vi "attribute_write_double.vi"(5 "Repeated Capability":string, 7 "Attribute":T1={"Identifier"="", "Descriptive name"="", "Data Type"=enum."Integer 32", "Command"="", "Access"=2, "Range Table"="", "Read Callback"="", "Write Callback"="", "Range Callback"="", "Check Callback"="", "Rngtable Callback"="", "Coerce Callback"="", "Supported Models"="", "Instrument Options"="", "Repeated Capabilities"="", "Check Status Callback"="", "Index"=0, "Flag: OPC Wait"=FALSE, "Flag: Dont check status"=FALSE, "Flag: Cache Only"=FALSE} {"Access" items=["Read Only", "Write Only", "Read/Write"]}, 8 "error in":errorcluster, 10 "double in":dbl, 11 "VISA resource name":refnum<visa-resource-name>) -> (0 "error out":errorcluster, 3 "VISA resource name out":refnum<visa-resource-name>)   [LabVIEW 2014, in "rszvl_rsidr_core.lvlib"]
uses:
  rszvl_rsidr_core.lvlib
  type_Attribute.ctl
  type_Attribute_Data_Type.ctl
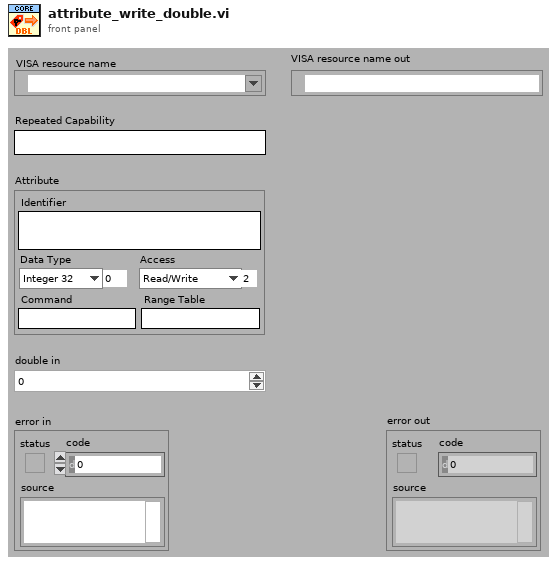
[diagram p1: front panel]
types:
  T1 = typedef "rszvl_rsidr_core.lvlib/type_Attribute.ctl" = cluster{"Identifier":string, "Descriptive name":string, "Data Type":T2, "Command":string, "Access":u16, "Range Table":string, "Read Callback":string, "Write Callback":string, "Range Callback":string, "Check Callback":string, "Rngtable Callback":string, "Coerce Callback":string, "Supported Models":string, "Instrument Options":string, "Repeated Capabilities":string, "Check Status Callback":string, "Index":i32, "Flag: OPC Wait":bool, "Flag: Dont check status":bool, "Flag: Cache Only":bool}
  T2 = typedef "rszvl_rsidr_core.lvlib/type_Attribute_Data_Type.ctl" = enum16{"Integer 32", "Double", "String", "Boolean", "None", "Integer 64"}
  T3 = typedef "rszvl_rsidr_core.lvlib/type_Session_Data.ctl" = cluster{"Instr type":string, "Instr type for err. msg.":string, "Installed Options":string[], "OPC Timeout":i32, "Query Instrument Status":bool, "Check Range":bool, "Check Options":bool, "Add LF to Write":bool, "Simulate":bool, "Logging":bool, "Logging params":variant, "Interface Type":enum16{"Unknown", "GPIB", "VXI", "GPIB_VXI", "ASRL", "PXI", "TCPIP", "USB", "SOCKET"}, "Fast Sweep":i32, "AdditionalFlags":i32, "WaitBeforeWrite":i32, "WaitBeforeRead":i32, "BinDataChunkSize":i64}
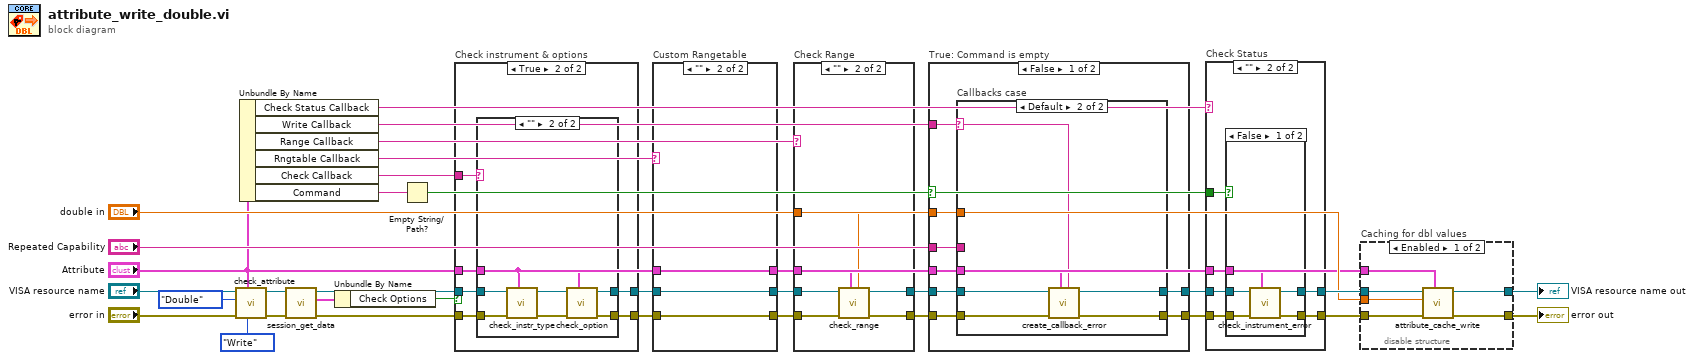
[diagram p0: block diagram]
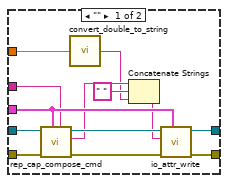
[diagram p2: hidden frame]
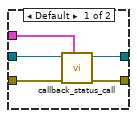
[diagram p4: hidden frame]
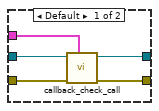
[diagram p7: hidden frame]
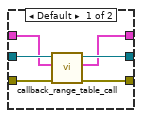
[diagram p8: hidden frame]
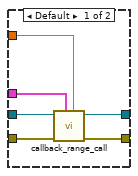
[diagram p9: hidden frame]
diagram:
  n1 = call "check_attribute.vi"("Access"=enum16{"Read", "Write"}."Write", "Attribute"="Attribute", "error in"="error in", "Data Type"=type_Attribute_Data_Type."Double", "VISA resource name"="VISA resource name") -> ("error out"=w9:errorcluster, "VISA resource name out"=w10:refnum<visa-resource-name>)  [unwired: 5 in]
  n2 = Unbundle By Name("Attribute") -> ("Check Status Callback"=w11:string, "Write Callback"=w12:string, "Range Callback"=w14:string, "Rngtable Callback"=w15:string, "Check Callback"=w13:string, "Command"=w1:string)
  n3 = call "session_get_data.vi"("error in"=w9, "VISA resource name"=w10) -> ("error out"=w7:errorcluster, "Session User Data out"=w4:T3, "VISA resource name out"=w8:refnum<visa-resource-name>)  [unwired: 7 in]
  n4 = Unbundle By Name(w4) -> ("Check Options"=w3:bool)
  n5 = Empty String/Path?(string/path=w1) -> (empty?=w33:bool)
  n6 = case "Check instrument & options" shown="True" w3 {
    tunnel: [w35 w41] -> w21
    tunnel: [w34 w40] -> w20
    tunnel: "Attribute" -> [_ w39]
    tunnel: w13 -> [_ w38]
    tunnel: w8 -> [w35 w37]
    tunnel: w7 -> [w34 w36]
    frame False {
    }
    frame True {
      n7 = case shown="\"\"" w38 {
        tunnel: [w45 w51] -> w41
        tunnel: [w43 w50] -> w40
        tunnel: w36 -> [w44 w49]
        tunnel: w39 -> [w42 w47]
        tunnel: w37 -> [w46 w48]
        frame Default {
          n8 = call "callback_check_call.vi"("Attribute"=w42, "error in"=w44, "VISA resource name"=w46) -> ("error out"=w43:errorcluster, "VISA resource name out"=w45:refnum<visa-resource-name>)  [unwired: 7 in]
        }
        frame "" {
          n9 = call "check_instr_type.vi"("Attribute"=w47, "error in"=w49, "VISA resource name"=w48) -> ("error out"=w53:errorcluster, "VISA resource name out"=w52:refnum<visa-resource-name>)  [unwired: 6 in, 1 out]
          n10 = call "check_option.vi"("Attribute"=w47, "error in"=w53, "VISA resource name"=w52) -> ("error out"=w50:errorcluster, "VISA resource name out"=w51:refnum<visa-resource-name>)  [unwired: 7 in]
        }
      }
    }
  }
  n11 = case "Custom Rangetable" shown="\"\"" w15 {
    tunnel: w21 -> [w59 w62]
    tunnel: w20 -> [w56 w61]
    tunnel: [w58 w62] -> w19
    tunnel: [w57 w61] -> w18
    tunnel: "Attribute" -> [w55 w60]
    tunnel: [w54 w60] -> w6
    frame Default {
      n12 = call "callback_range_table_call.vi"("error in"=w56, "Attribute in"=w55, "VISA resource name"=w59) -> ("error out"=w57:errorcluster, "Attribute out"=w54:T1, "VISA resource name out"=w58:refnum<visa-resource-name>)  [unwired: 6 in]
    }
    frame "" {
    }
  }
  n13 = case "Check Range" shown="\"\"" w14 {
    tunnel: w19 -> [w68 w74]
    tunnel: w18 -> [w65 w73]
    tunnel: w6 -> [w63 w70]
    tunnel: [w66 w72] -> w23
    tunnel: [w67 w71] -> w22
    tunnel: "double in" -> [w64 w69]
    frame Default {
      n14 = call "callback_range_call.vi"("Attribute Value"=w64, "Attribute"=w63, "error in"=w65, "VISA resource name"=w68) -> ("error out"=w66:errorcluster, "VISA resource name out"=w67:refnum<visa-resource-name>)  [unwired: 4 in, 2 out]
    }
    frame "" {
      n15 = call "check_range.vi"("Attribute Value"=w69, "Attribute"=w70, "error in"=w73, "VISA resource name"=w74) -> ("error out"=w72:errorcluster, "VISA resource name out"=w71:refnum<visa-resource-name>)  [unwired: 4 in, 2 out]
    }
  }
  n16 = case "True: Command is empty" shown="False" w33 {
    tunnel: "Repeated Capability" -> [w82 _]
    tunnel: w23 -> [w81 w102]
    tunnel: w22 -> [w80 w103]
    tunnel: "double in" -> [w79 _]
    tunnel: w6 -> [w78 _]
    tunnel: [w77 w103] -> w17
    tunnel: [w76 w102] -> w16
    tunnel: w12 -> [w75 _]
    frame False {
      n17 = case "Callbacks case" shown="Default" w75 {
        selector: w75 -> [_ w96]
        tunnel: w80 -> [w94 w100]
        tunnel: w81 -> [w92 w101]
        tunnel: w82 -> [w88 _]
        tunnel: [w91 w98] -> w77
        tunnel: [w90 w99] -> w76
        tunnel: w78 -> [w89 w97]
        tunnel: w79 -> [w83 _]
        frame "" {
          n18 = call "rep_cap_compose_cmd.vi"("Repeated Capability"=w88, "Attribute"=w89, "error in"=w92, "VISA resource name"=w94) -> ("error out"=w93:errorcluster, "Command out"=w87:string, "VISA resource name out"=w95:refnum<visa-resource-name>)  [unwired: 5 in]
          n19 = call "convert_double_to_string.vi"("double in"=w83) -> ("string out"=w84:string)  [unwired: 4 in]
          n20 = Concatenate Strings(w87, " " ("string"), w84) -> (w85:string)
          n21 = call "io_attr_write.vi"("Attribute"=w89, "error in"=w93, "write buffer"=w85, "VISA resource name"=w95) -> ("error out"=w90:errorcluster, "VISA resource name out"=w91:refnum<visa-resource-name>)  [unwired: 6 in]
        }
        frame Default {
          n22 = call "create_callback_error.vi"("Callback Name"=w96, "Attribute"=w97, "error in"=w101, "VISA resource name"=w100) -> ("error out"=w99:errorcluster, "VISA resource name out"=w98:refnum<visa-resource-name>)  [unwired: 6 in]
        }
      }
    }
    frame True {
    }
  }
  n23 = case "Check Status" shown="\"\"" w11 {
    tunnel: w16 -> [w108 w113]
    tunnel: [w107 w112] -> w32
    tunnel: [w106 w111] -> w31
    tunnel: w17 -> [w105 w114]
    tunnel: w6 -> [w104 w110]
    tunnel: w33 -> [_ w109]
    frame Default {
      n24 = call "callback_status_call.vi"("Attribute"=w104, "error in"=w108, "VISA resource name"=w105) -> ("error out"=w107:errorcluster, "VISA resource name out"=w106:refnum<visa-resource-name>)  [unwired: 7 in]
    }
    frame "" {
      n25 = case shown="False" w109 {
        tunnel: w114 -> [w119 w121]
        tunnel: w113 -> [w118 w120]
        tunnel: [w117 w120] -> w112
        tunnel: [w116 w121] -> w111
        tunnel: w110 -> [w115 _]
        frame False {
          n26 = call "check_instrument_error.vi"("Attribute"=w115, "error in"=w118, "VISA resource name"=w119) -> ("error out"=w117:errorcluster, "VISA resource name out"=w116:refnum<visa-resource-name>)  [unwired: 7 in]
        }
        frame True {
        }
      }
    }
  }
  n27 = disable-structure "Caching for dbl values" shown="Enabled" {
    disable-tunnel: [w127 w129] -> w27
    disable-tunnel: [w126 w128] -> w26
    disable-tunnel: w32 -> [w125 w128]
    disable-tunnel: w31 -> [w124 w129]
    disable-tunnel: "double in" -> [w123 _]
    disable-tunnel: "Attribute" -> [w122 _]
    frame Enabled {
      n28 = call "attribute_cache_write.vi"("Attribute"=w122, "error in"=w125, "Value in"=w123, "VISA resource name"=w124) -> ("error out"=w126:errorcluster, "VISA resource name out"=w127:refnum<visa-resource-name>)  [unwired: 6 in]
    }
    frame Disabled {
    }
  }
  "error out" <- w26
  "VISA resource name out" <- w27
